vi "(SubVI) Calculate xDNA for Passive Force Clamp Data_YCC.vi"(4 "conversion factor (V/um)":dbl, 5 "Start point of Xbd for pFC (nm)":dbl, 6 "Move to (um)":dbl, 7 "trap height(nm)":dbl, 8 "QPD center value (V)":dbl, 9 "Stage center point (um)":dbl, 10 "Target QPD radius (nm)":dbl=500.0, 11 "QPD Array (V)":dbl[](array[numeric])) -> (0 "Check Xbd for pFC (nm)":dbl, 1 "zbd (nm)":dbl[](array[numeric]), 3 "xDNA (nm)":dbl[](array[numeric]))   [LabVIEW 2014]
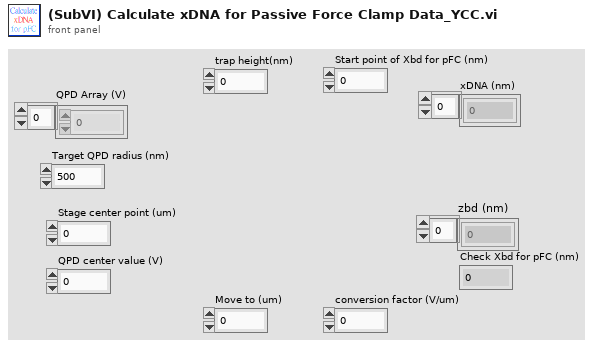
[diagram p1: front panel]
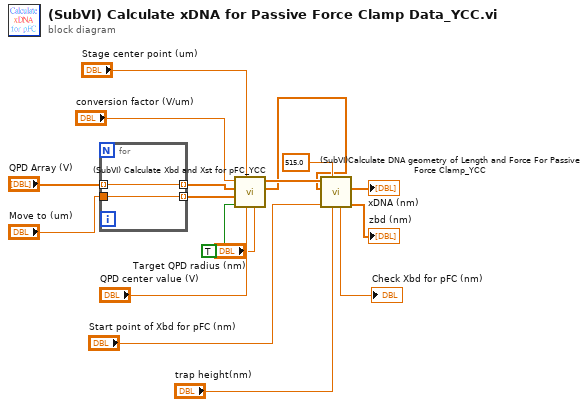
[diagram p0: block diagram]
diagram:
  n1 = for {
    tunnel: "QPD Array (V)" -> [w18] mode=indexing
    tunnel: [w19] -> w14 mode=indexing
    tunnel: "Move to (um)" -> [w19]
    tunnel: [w18] -> w13 mode=indexing
  }
  n2 = call "(SubVI) Calculate Xbd and Xst for pFC_YCC.vi"("Target QPD radius (nm)"="Target QPD radius (nm)", "Target QPD (V)"="QPD center value (V)", "cr"="Stage center point (um)", "X=T\nY=F"=TRUE ("X=T\nY=F"), "Stage Position"=w14, "QPD signal"=w13, "conversion factor (V/um)"="conversion factor (V/um)") -> ("Xst (nm)"=w1:dbl[], "Xbd (nm)"=w9:dbl[])  [unwired: 3 in]
  n3 = call "(SubVI)Calculate DNA geometry of Length and Force For Passive Force Clamp_YCC.vi"("trap height(nm)"="trap height(nm)", "bead radius(nm)"=515.0, "Start point of Xbd for pFC (nm)"="Start point of Xbd for pFC (nm)", "Xst (nm)"=w1, "Xbd (nm)"=w9) -> ("zbd (nm)"=→"zbd (nm)":dbl[], "xDNA (nm)"=→"xDNA (nm)":dbl[], "Check Xbd for pFC (nm)"=→"Check Xbd for pFC (nm)":dbl)  [unwired: 4 in]
